vi "time.elapse.vi"(3 "Set Time":dbl) -> ()   [LabVIEW 2015]
doc: "This VI acquires non-waveform data (a random number between 0 and 1) at every iteration of the loop and bundles it with the corresponding timestamp when it was acquired. The cluster of x-array data and y-array data are passed to an XY Graph, which plots the data points vs. their corresponding timestamps."
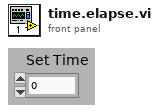
[diagram p1: front panel]
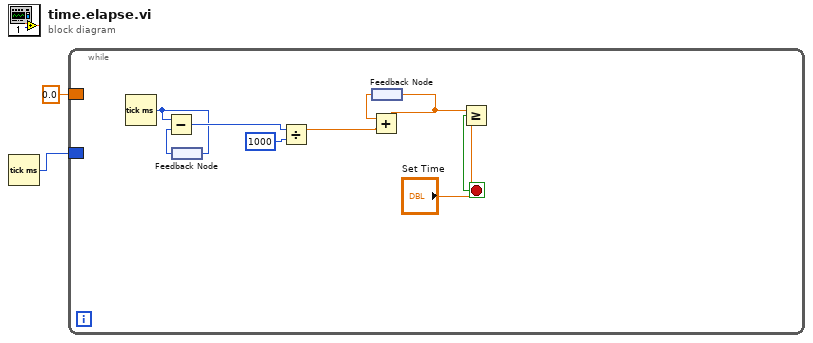
[diagram p0: block diagram]
diagram:
  n1 = Tick Count (ms)() -> (millisecond timer value=w1:u32)
  n2 = while {
    border: 0.0 -> [_]
    border: w1 -> [_]
    stop <- w3 stop-if-true
    n3 = Tick Count (ms)() -> (millisecond timer value=w8:u32)
    n4 = feedback-in #1(w8) -> ()
    n5 = feedback #1() -> (w9:u32)
    n6 = Subtract(x=w8, y=w9) -> (x-y=w10:u32)
    n7 = Divide(x=w10, y=u32 1000) -> (x/y=w7:dbl)
    n8 = feedback #2() -> (w6:dbl)
    n9 = Add(x=w6, y=w7) -> (x+y=w5:dbl)
    n10 = feedback-in #2(w5) -> ()
    n11 = Greater Or Equal?(x=w5, y="Set Time") -> (x >= y?=w3:bool)
    n12 = Wait Until Next ms Multiple(millisecond multiple=u32 10) -> ()  [unwired: 1 out]
  }
